vi "习题7.2.vi"() -> ()   [LabVIEW 2017]
panel:
  out "波形图":cluster{dbl[]}[](graph)
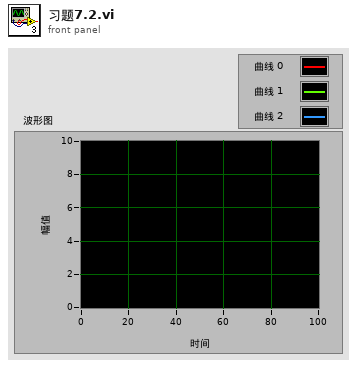
[diagram p1: front panel]
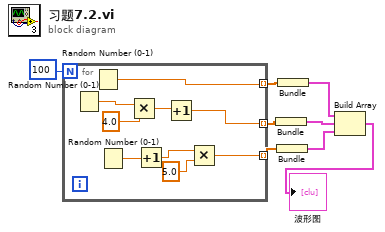
[diagram p0: block diagram]
diagram:
  n1 = for {
    N: 100 -> [_]
    tunnel: [w17] -> w7 mode=indexing
    tunnel: [w13] -> w6 mode=indexing
    tunnel: [w9] -> w5 mode=indexing
    n2 = Random Number (0-1)() -> (number: 0 to 1=w15:dbl)
    n3 = Random Number (0-1)() -> (number: 0 to 1=w17:dbl)
    n4 = Random Number (0-1)() -> (number: 0 to 1=w12:dbl)
    n5 = Multiply(x=w15, y=4.0) -> (x*y=w16:dbl)
    n6 = Increment(x=w12) -> (x+1=w11:dbl)
    n7 = Increment(x=w16) -> (x+1=w13:dbl)
    n8 = Multiply(x=w11, y=5.0) -> (x*y=w9:dbl)
  }
  n9 = Bundle(w6) -> (w3:cluster{dbl[]})  [unwired: 1 in]
  n10 = Bundle(w5) -> (w2:cluster{dbl[]})  [unwired: 1 in]
  n11 = Bundle(w7) -> (w4:cluster{dbl[]})  [unwired: 1 in]
  n12 = Build Array(w4, w3, w2) -> (→"波形图":cluster{dbl[]}[])
